vi "Predict Pos from Encoders, Compass.vi"(7 "Cmd":enum16{"Init", "Run"}(ring), 8 "error in (no error)":errorcluster) -> (0 "error out":errorcluster, 2 "XYT":cluster{"X":dbl, "Y":dbl, "Theta":dbl})   [LabVIEW 2009]
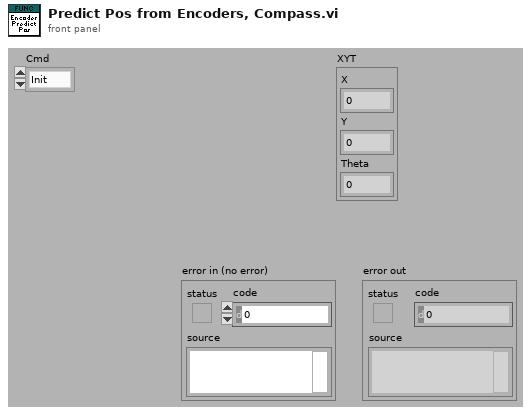
[diagram p1: front panel]
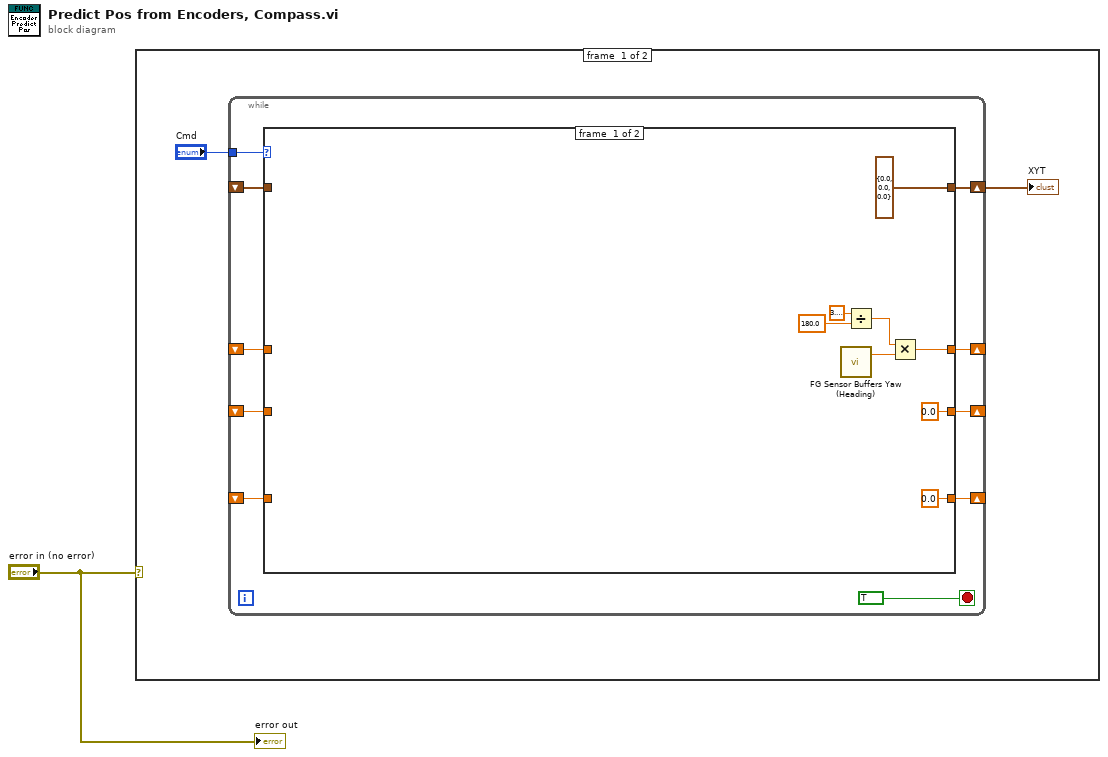
[diagram p0: block diagram]
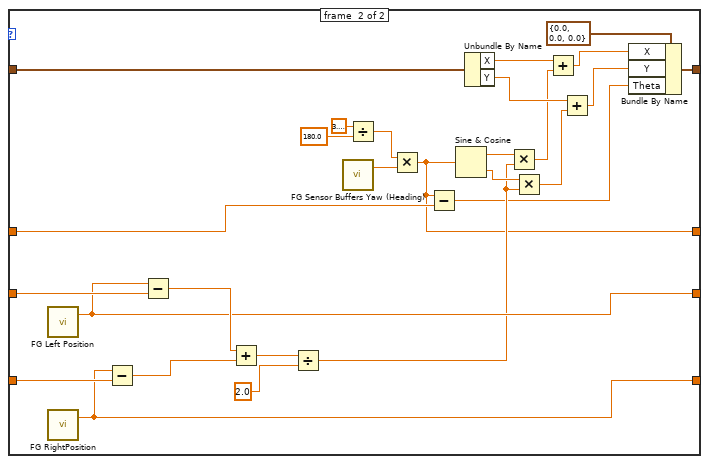
[diagram p2: hidden frame]
diagram:
  n1 = case shown="No Error" "error in (no error)" {
    frame #0 {
      n2 = while {
        shift-right: [w9] -> _
        shift-left: _ -> [w12]
        shift-right: [w10] -> _
        shift-left: _ -> [w11]
        shift-right: [w8] -> w2
        shift-left: _ -> [w13]
        tunnel: "Cmd" -> [w6]
        shift-right: [w5] -> _
        shift-left: _ -> [w4]
        stop <- TRUE stop-if-true
        n3 = case shown="\"Run\"" w6 {
          tunnel: w13 -> [_ w33]
          tunnel: w12 -> [_ w44]
          tunnel: w11 -> [_ w43]
          tunnel: [0.0 ("Right Dist Travelled Out (cm)") w37] -> w10
          tunnel: [0.0 ("Left Dist Travelled Out (cm)") w36] -> w9
          tunnel: [cluster{"X":dbl, "Y":dbl, "Theta":dbl} {"X"=0.0, "Y"=0.0, "Theta"=0.0} ("Cluster") w34] -> w8
          tunnel: [w15 w22] -> w5
          tunnel: w4 -> [_ w24]
          frame #0 {
            n4 = call "FG Sensor Buffers Yaw (Heading).vi"() -> ("Yaw Buffer Out"=w16:dbl)  [unwired: 3 in]
            n5 = Divide(x=3.141592653589793, y=180.0) -> (x/y=w17:dbl)
            n6 = Multiply(x=w17, y=w16) -> (x*y=w15:dbl)
          }
          frame #1 {
            n7 = call "FG Left Position.vi"() -> ("Left Dist Travelled Out (cm)"=w36:dbl)  [unwired: 3 in]
            n8 = call "FG RightPosition.vi"() -> ("Right Dist Travelled Out (cm)"=w37:dbl)  [unwired: 3 in]
            n9 = Subtract(x=w37, y=w43) -> (x-y=w45:dbl)
            n10 = Subtract(x=w36, y=w44) -> (x-y=w46:dbl)
            n11 = Add(x=w46, y=w45) -> (x+y=w48:dbl)
            n12 = Divide(x=w48, y=2.0) -> (x/y=w29:dbl)
            n13 = call "FG Sensor Buffers Yaw (Heading).vi"() -> ("Yaw Buffer Out"=w28:dbl)  [unwired: 3 in]
            n14 = Divide(x=3.141592653589793, y=180.0) -> (x/y=w38:dbl)
            n15 = Multiply(x=w38, y=w28) -> (x*y=w22:dbl)
            n16 = Subtract(x=w22, y=w24) -> (x-y=w23:dbl)
            n17 = Sine & Cosine(0:w22) -> (1:w42:dbl, 2:w41:dbl)
            n18 = Unbundle By Name(w33) -> ("X"=w32:dbl, "Y"=w31:dbl)
            n19 = Multiply(x=w42, y=w29) -> (x*y=w27:dbl)
            n20 = Multiply(x=w41, y=w29) -> (x*y=w26:dbl)
            n21 = Add(x=w32, y=w27) -> (x+y=w30:dbl)
            n22 = Add(x=w31, y=w26) -> (x+y=w35:dbl)
            n23 = Bundle By Name(cluster=cluster{"X":dbl, "Y":dbl, "Theta":dbl} {"X"=0.0, "Y"=0.0, "Theta"=0.0} ("Cluster"), "X"=w30, "Y"=w35, "Theta"=w23) -> (w34:cluster{"X":dbl, "Y":dbl, "Theta":dbl})
          }
        }
      }
      "XYT" <- w2
    }
    frame #1 {
    }
  }
  "error out" <- "error in (no error)"
